vi "Productor.vi"() -> ()   [LabVIEW 2020]
uses:
  Options.ctl
panel:
  out "Mouse encima\nde Boolean":bool
  in  "Boolean":bool
  out "Tiempo UE":timestamp
  in  "String":string
  in  "stop":bool
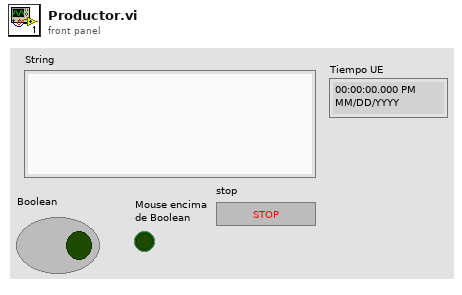
[diagram p1: front panel]
types:
  T1 = typedef "Options.ctl" = enum16{"Create", "Get", "Destroy"}
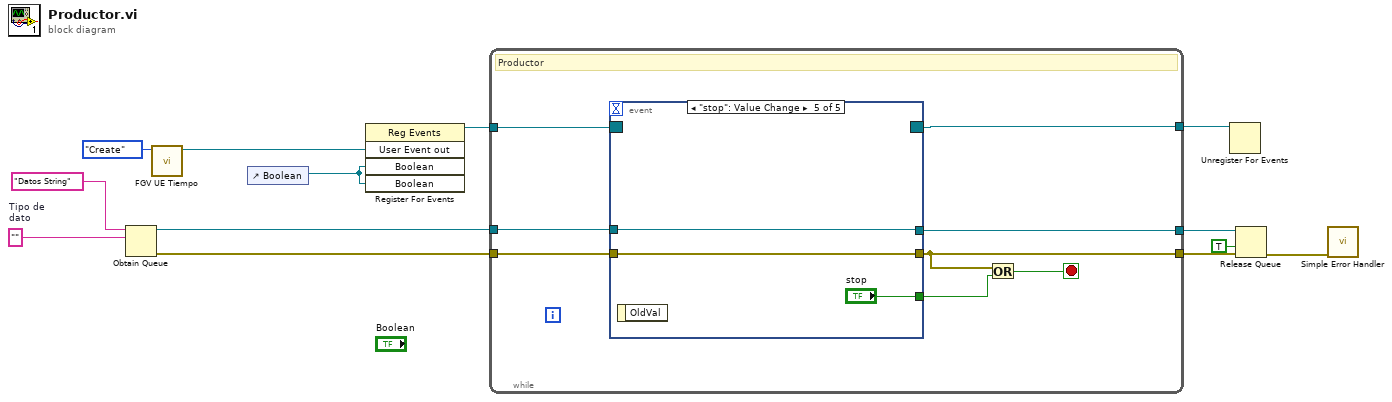
[diagram p0: block diagram]
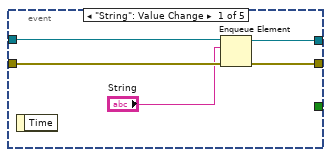
[diagram p2: hidden frame]
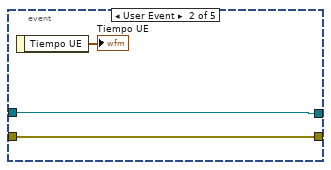
[diagram p3: hidden frame]
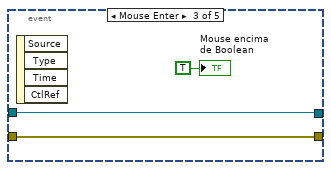
[diagram p4: hidden frame]
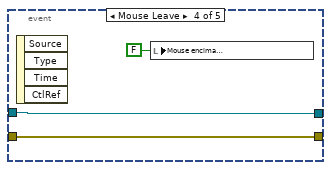
[diagram p5: hidden frame]
diagram:
  w12 = ""  # Tipo de dato
  n1 = Obtain Queue(name (unnamed)="Datos String", element data type=w12) -> (queue out=w8:refnum<queue>, error out=w13:errorcluster)  [unwired: 3 in, 1 out]
  n2 = call "FGV UE Tiempo.vi"("Enum"=Options."Create") -> ("User Event out"=w4:refnum<user-event>)  [unwired: 10 in]
  n3 = control-ref of="Boolean"() -> (w2:refnum<vi>)
  n4 = register-events(w4, w2, w2) -> (reference out=w5:refnum<event-registration>)  [unwired: 2 in, 1 out]
  n5 = while {
    tunnel: w8 -> [w21]
    tunnel: w13 -> [w20]
    tunnel: [w18] -> w11
    tunnel: [w17] -> w10
    tunnel: w5 -> [w15]
    tunnel: [w14] -> w3
    stop <- w19 stop-if-true
    # "Productor"
    n6 = event shown="[4] \"stop\": Value Change" {
      selector: w15 -> [_ _ _ _ _]
      dyn-events: [_ _ _ _ _] -> w14
      timeout: _ -> [_ _ _ _ _]
      tunnel: w21 -> [w26 w29 w32 w35 w37]
      tunnel: w20 -> [w25 w28 w31 w34 w36]
      tunnel: [w24 w28 w31 w34 w36] -> w18
      tunnel: [w23 w29 w32 w35 w37] -> w17
      tunnel: [_ _ _ _ "stop"] -> w16
      event "String": Value Change {
        n7 = event-data() -> ()  [unwired: 1 in, 1 out]
        n8 = Enqueue Element(queue=w26, element="String", error in (no error)=w25) -> (queue out=w23:refnum<queue>, error out=w24:errorcluster)  [unwired: 1 in, 1 out]
      }
      event User Event {
        n9 = event-data() -> ("Tiempo UE"=→"Tiempo UE":timestamp)  [unwired: 1 in]
      }
      event Mouse Enter {
        n10 = event-data() -> ()  [unwired: 1 in, 4 out]
        "Mouse encima\nde Boolean" <- TRUE ("Mouse encima\nde Boolean")
      }
      event Mouse Leave {
        n11 = event-data() -> ()  [unwired: 1 in, 4 out]
        n12 = local write "Mouse encima\nde Boolean"(FALSE ("Mouse encima\nde Boolean")) -> ()
      }
      event "stop": Value Change {
        n13 = event-data() -> ()  [unwired: 1 in, 1 out]
      }
    }
    n14 = Or(x=w18, y=w16) -> (x .or. y?=w19:bool)
  }
  n15 = Unregister For Events(event registration refnum=w3) -> ()  [unwired: 1 in, 1 out]
  n16 = Release Queue(queue=w10, force destroy? (F)=TRUE, error in (no error)=w11) -> (error out=w9:errorcluster)  [unwired: 2 out]
  n17 = call <vilib>:"Simple Error Handler.vi"("error in (no error)"=w9) -> ()  [unwired: 4 in, 5 out]
